vi "input.vi"(8 "error in":errorcluster, 10 "input allocation":T1, 11 "ActiveFrontEndModule runtime in":refnum<class "ActiveFrontEndModule runtime.lvclass">) -> (0 "error out":errorcluster, 2 "input data":T1, 3 "ActiveFrontEndModule runtime out":refnum<class "ActiveFrontEndModule runtime.lvclass">)   [LabVIEW 2017, in "ActiveFrontEndModule runtime.lvclass"]
doc: "Provides an interface for reading data from a module at runtime. While this interface performs no operations, a child should provide an override which may read from any open sessions, references, or interfaces."
uses:
  ActiveFrontEndModule runtime.lvclass
  <vilib>/NI/Tag Bus/table/data table.ctl
  ActiveFrontEndModule runtime.lvclass/ActiveFrontEndModule runtime.ctl
  input user data.ctl
  <vilib>/NI/PowerElectronicsControl/ActiveFrontEnd/AFE_Interface/AFE_interface.lvlib
  <vilib>/NI/Tag Bus/table/data table.lvlib
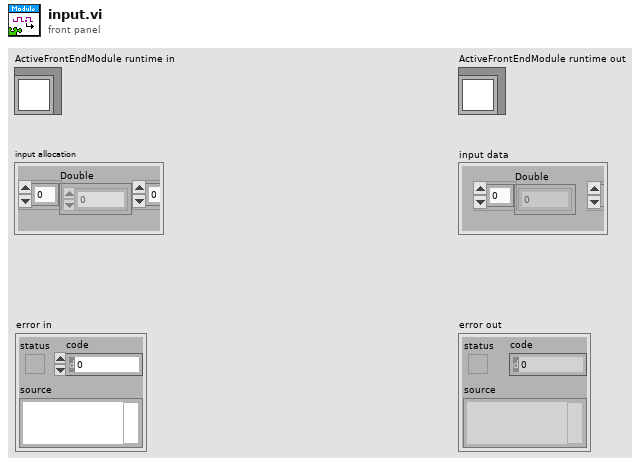
[diagram p1: front panel]
types:
  T1 = typedef "tag bus.lvlib/data table.lvlib/data table.ctl" = cluster{"Double":dbl[], "Single":sgl[], "I64":i64[], "I32":i32[], "I16":i16[], "I8":i8[], "U64":u64[], "U32":u32[], "U16":u16[], "U8":u8[], "Boolean":bool[], "String":string[], "Array of Double":cluster{"DBL Array":dbl[]}[], "Array of Single":cluster{"SGL Array":sgl[]}[], "Array of I64":cluster{"I64 Array":i64[]}[], "Array of I32":cluster{"I32 Array":i32[]}[], "Array of I16":cluster{"I16 Array":i16[]}[], "Array of I8":cluster{"I8 Array":i8[]}[], "Array of U64":cluster{"U64 Array":u64[]}[], "Array of U32":cluster{"U32 Array":u32[]}[], "Array of U16":cluster{"U16 Array":u16[]}[], "Array of U8":cluster{"U8 Array":u8[]}[], "Array of Boolean":cluster{"Boolean Array":bool[]}[], "Array of String":cluster{"String Array":string[]}[]}
  T2 = typedef "ActiveFrontEndModule runtime.lvclass/input user data.ctl" = cluster{"AFE_VDCLink":dbl, "AFE_P":dbl, "AFE_Q":dbl, "AFE_pf":dbl}
  T3 = typedef "ActiveFrontEndModule configuration.lvclass/input data indices.ctl" = cluster{"Double.AFE_VDCLink":i32, "Double.AFE_P":i32, "Double.AFE_Q":i32, "Double.AFE_pf":i32}
  T4 = typedef "AFE_interface.lvlib/InterfaceRef.ctl" = cluster{"instruction target":refnum<class "niInstr Instruction Target v1 Host.lvclass">, "context":refnum<class "niInstr Instruction Framework Context v1 Host.lvclass">}
  T5 = typedef "AFE_interface.lvlib/Feedback.ctl" = cluster{"VDClink":dbl, "P":dbl, "Q":dbl, "pf":dbl}
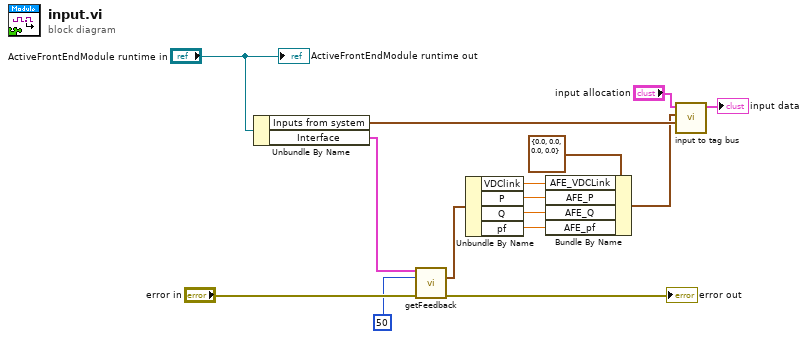
[diagram p0: block diagram]
diagram:
  n1 = Unbundle By Name("ActiveFrontEndModule runtime in") -> ("Inputs from system"=w12:T3, "Interface"=w9:T4)
  n2 = call <vilib>:"getFeedback.vi"("Interface in"=w9, "timeout (5000 ms)"=50, "error in"="error in") -> ("feedback"=w5:T5, "error out"=→"error out":errorcluster)  [unwired: 10 in, 1 out]
  n3 = Unbundle By Name(w5) -> ("VDClink"=w4:dbl, "P"=w3:dbl, "Q"=w2:dbl, "pf"=w1:dbl)
  n4 = Bundle By Name(cluster=T2 {"AFE_VDCLink"=0.0, "AFE_P"=0.0, "AFE_Q"=0.0, "AFE_pf"=0.0} ("data cluster"), "AFE_VDCLink"=w4, "AFE_P"=w3, "AFE_Q"=w2, "AFE_pf"=w1) -> (w6:T2)
  n5 = call "input to tag bus.vi"("indices"=w12, "data cluster"=w6, "tag bus in"="input allocation") -> ("tag bus out"=→"input data":T1)  [unwired: 8 in]
  "ActiveFrontEndModule runtime out" <- "ActiveFrontEndModule runtime in"
